vi "Read Config From File.vi"(8 "error in (no error)":errorcluster, 11 "System in":refnum<class "System.lvclass">) -> (0 "error out":errorcluster, 2 "Config As String":string, 3 "System out":refnum<class "System.lvclass">)   [LabVIEW 2013, in "System.lvclass"]
uses:
  System.lvclass
  System.lvclass/System.ctl
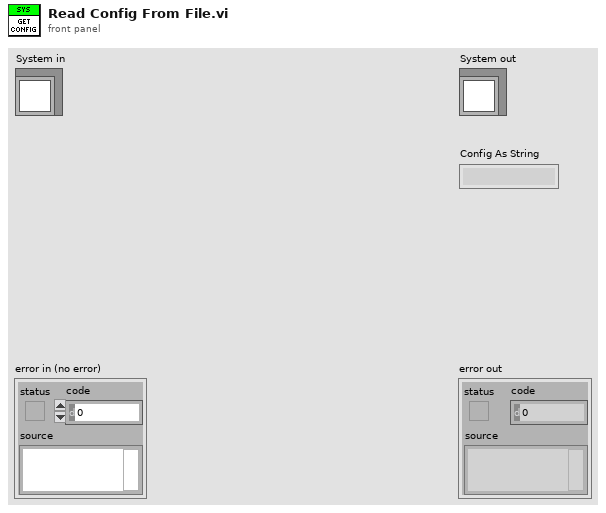
[diagram p1: front panel]
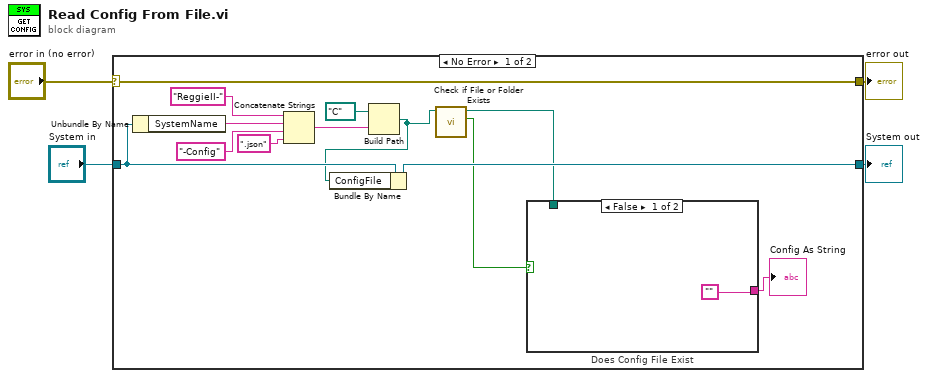
[diagram p0: block diagram]
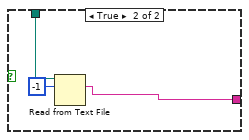
[diagram p2: hidden frame]
diagram:
  n1 = case shown="No Error" "error in (no error)" {
    selector: "error in (no error)" -> [w17 w23]
    tunnel: [w17 w23] -> w3
    tunnel: [w9 w22] -> w1
    tunnel: "System in" -> [w16 w22]
    frame No Error {
      n2 = Unbundle By Name(w16) -> ("SystemName"=w14:string)
      n3 = Concatenate Strings("ReggieII-" ("string"), w14, "-Config" ("string"), ".json" ("string")) -> (w11:string)
      n4 = Build Path(base path=path "C:/", name or relative path=w11) -> (appended path=w8:path)
      n5 = Bundle By Name(cluster=w16, "ConfigFile"=w8) -> (w9:refnum<class "System.lvclass">)
      n6 = call <vilib>:"Check if File or Folder Exists.vi"("path"=w8) -> ("file or folder exists?"=w7:bool, "dup path"=w6:path)  [unwired: 8 in, 1 out]
      n7 = case "Does Config File Exist" shown="False" w7 {
        tunnel: w6 -> [_ w21]
        tunnel: ["" w19] -> w5
        frame False {
        }
        frame True {
          n8 = Read from Text File(file (use dialog)=w21, count=-1) -> (text=w19:string)  [unwired: 2 in, 3 out]
        }
      }
      "Config As String" <- w5
    }
    frame Error {
    }
  }
  "error out" <- w3
  "System out" <- w1
